vi "16chaneffective.vi"() -> ()   [LabVIEW 2013]
doc: "Cont(inuous) Acq(uire) & Chart (hw timed) demonstrates the hardware timed, non-buffered technique of data acquisition. The scan clock on the board controls acquisition timing. Acquired scans are read directly from the device's FIFO using AI Single Scan. \n\nThe acquisition is configured with no buffer, and the on-board scan clock started at the selected scan rate. In the first loop iteration, the newest (most recent) scan is read from the FIFO. In each subsequent loop iteration AI Single Scan is called to read the oldest scan from the FIFO. Then if a scan is missed because the acquisition does not keep up, an error message will be displayed, and the acquisition stopped. Each scan is plotted on the chart after it is read. \n\nA common reason to use non-buffered acquisition is that some kind of processing needs to be done for each data point. You will probably want to add more functions to the diagram to customize this VI for your application. The acquisition rate you can achieve depends on how much processing and display the VI must do. This VI calls a subVI named My Single-Scan Processing. Add whatever processing you need to this subVI, or replace it with one of your own. The data processing subVI also demonstrates how to use error clusters in your own subVIs, so they can be included in the error data flow chain.\n\nBefore running this VI, set the values of the controls on the front panel. Select Show Help Window from the Help menu to see a description of each control. If the values you select for all the controls are values you will usually use, select Make Current Values Default from the Operate menu and save the VI. Or, you may save individual control's default values by popping up on the control, selecting Data Operations, then selecting Make Current Value Default, and saving the VI."
uses:
  <vilib>/Utility/error.llb/DialogType.ctl
  <vilib>/DAQmx/read.llb/DAQmx Read (Analog 2D DBL NChan NSamp).vi
  BiaxGlobals (16chan).vi
  <vilib>/DAQmx/create/channels.llb/DAQmx Create Channel (AI-Voltage-Basic).vi
  <vilib>/DAQmx/configure/timing.llb/DAQmx Timing (Sample Clock).vi
  <vilib>/DAQmx/configure/trigger.llb/DAQmx Start Trigger (Digital Edge).vi
  effectiveglobals.vi
  <vilib>/DAQmx/miscellaneous.llb/DAQmx Fill In Error Info.vi
  <resource>/objmgr/daqmx.rc
panel:
  in  "Show plot":bool
  out "Zero Voltage Y":dbl
  in  "Calibration y-axis (V/unit)":dbl=1.0 format="%#_6f"
  in  "Select y-axis":string(combo)="Porosity"
  in  "Calibration x-axis (V/unit)":dbl=1.0 format="%#_6f"
  in  "Select x-axis":string(combo)="Time (s)"
  out "Offset Voltage 2":dbl
  out "Offset Voltage 1":dbl
  in  "Offset X-axis 2":bool
  in  "Offset X-axis 1":bool
  in  "Zero y-axis":bool
  out "XY plot":cluster{"Y":dbl[], "Y":dbl[]}[](graph)
  in  "Reset plot":bool
  out "Zero Voltage X":dbl
  in  "Zero X-axis":bool
  out "Porosity (%)":dbl format="%_4f"
  in  "Material density (g/cm3)":dbl=2.17
  in  "Amount of material (g)":dbl=42.88 format="%_4f"
  in  "Thickness (2 layers, mm)":dbl=11.28 format="%_4f"
  in  "Zero Hor DCDT":bool
  out "Average Pore pressure":dbl=0.0015205308
  out "Zeroed at:":i32
  out "Zero Voltage":dbl format="%_6g"
  in  "Zero Pore pressure A":bool
  out "Zeroed at:":i32
  out "Zero Voltage":dbl format="%_6g"
  in  "Zero Pore pressure B":bool
  out "Effective normal \nstress (MPa)":dbl=0.0015205308
  in  "Sample\n Area (m2)":dbl=0.003078
  out "Zeroed at:":i32
  out "Zero Voltage":dbl format="%_6g"
  in  "Zero Confine":bool
  in  "Horizontal Load":bool=TRUE
  out "Zeroed at:":i32
  out "Zero Voltage":dbl format="%_6g"
  in  "Zero Normal":bool
  out "Array 2":i32[][](array[numeric])=[[10000, 0, -17, -1030, -696, -422, -1063, -1097, -410, -661, -1080]]
  out "AUX8 (ch11)":dbl format="%.4f"
  out "AUX7 (ch10)":dbl format="%.4f"
  out "AUX6 (ch9)":dbl format="%.4f"
  out "AUX5 (ch8)":dbl format="%.4f"
  out "AUX4 (ch7)":dbl format="%.4f"
  out "AUX3 (ch6)":dbl format="%.4f"
  out "AUX2 (ch5)":dbl format="%.4f"
  out "AUX1 (ch4)":dbl format="%.4f"
  out "Hor Load (ch0)":dbl format="%.4f"
  out "Vert Load (ch2)":dbl format="%.4f"
  out "Hor LVDT":dbl format="%.4f"
  out "Vert LVDT (ch3)":dbl format="%.4f"
  out "Array 17":i32[][](array[numeric])=[[10000, -673, -5, -1015, -683, -421, -1049, -1100, -413, -693, -1121]]
  out "Array 16":i32[][](array[numeric])=[[10000, -673, -5, -1015, -683, -421, -1049, -1100, -413, -693, -1121]]
  out "Array 15":i32[][](array[numeric])=[[10000, -673, -5, -1015, -683, -421, -1049, -1100, -413, -693, -1121]]
  out "Array 14":i32[][](array[numeric])=[[10000, -685, -5, -1012, -680, -418, -1052, -1092, -421, -673, -1097]]
  out "AUX12 (ch15)":dbl format="%.4f"
  out "AUX11 (ch14)":dbl format="%.4f"
  out "AUX10 (ch13)":dbl format="%.4f"
  out "AUX9 (ch12)":dbl format="%.4f"
  out "element 15":string
  out "element 14":string
  out "element 13":string
  out "element 12":string
  out "element 11":string
  out "element 10":string
  out "element 9":string
  out "element 8":string
  out "element 7":string
  out "element 6":string="  "
  out "element 5":string
  out "element 4":string
  out "element 3":string
  out "element 2":string
  out "element":string
  out "element":string
  out "Stress-strain-temp vs time (Voltage)":dbl[][](graph)
  out "Array 13":i32[][](array[numeric])
  out "Array 12":i32[][](array[numeric])
  out "Array 11":i32[][](array[numeric])
  out "Array 10":i32[][](array[numeric])
  out "Array 9":i32[][](array[numeric])
  out "Array 8":i32[][](array[numeric])
  out "Array 7":i32[][](array[numeric])
  out "Array 6":i32[][](array[numeric])
  out "Array 5":i32[][](array[numeric])
  out "Array 4":i32[][](array[numeric])
  out "Array 3":i32[][](array[numeric])
  out "Array":i32[][](array[numeric])
  out "10000":bool
  in  "10 kHz":bool
  out "Processor scan rate":i32
  out "Present sample number":i32
  in  "1 Hz":bool
  out "1":bool
  out "10":bool
  out "100":bool
  out "1000":bool
  in  "10 Hz":bool
  in  "100 Hz":bool
  in  "1000 Hz":bool
  out "Data Recording Rate":i32(slide) scale=1.0..10000.0
  out "Write interval":i32
  out "Write countdown":i32
  out "Time into data acq. (s)":i32
  out "Saved sample No.":i32
  out "Record rate (samp/s)":i32
  out "No. of scans in backlog":i32
  in  "stop":bool
  # "Input Signals (volts)"
  # "To File (24 bit)"
  # "S\nI\nG\nN\nA\nL\n\nV\nO\nL\nT\nA\nG\nE"
  # "Timestamp"
  # "Data Recording Info"
  # "Acquisition Statistics"
  # "Sample (point) Number"
  # "Low gain"
  # "High gain"
  # "NOTE:  This instrument will write data (time channel then Channels 0-15) to a user defined filename.  The file is written in binary format without a header. The time channel is comprised of numbers indicating the data recording frequency (eg 1, 10, 100, 1000, 10000  samples per second)."
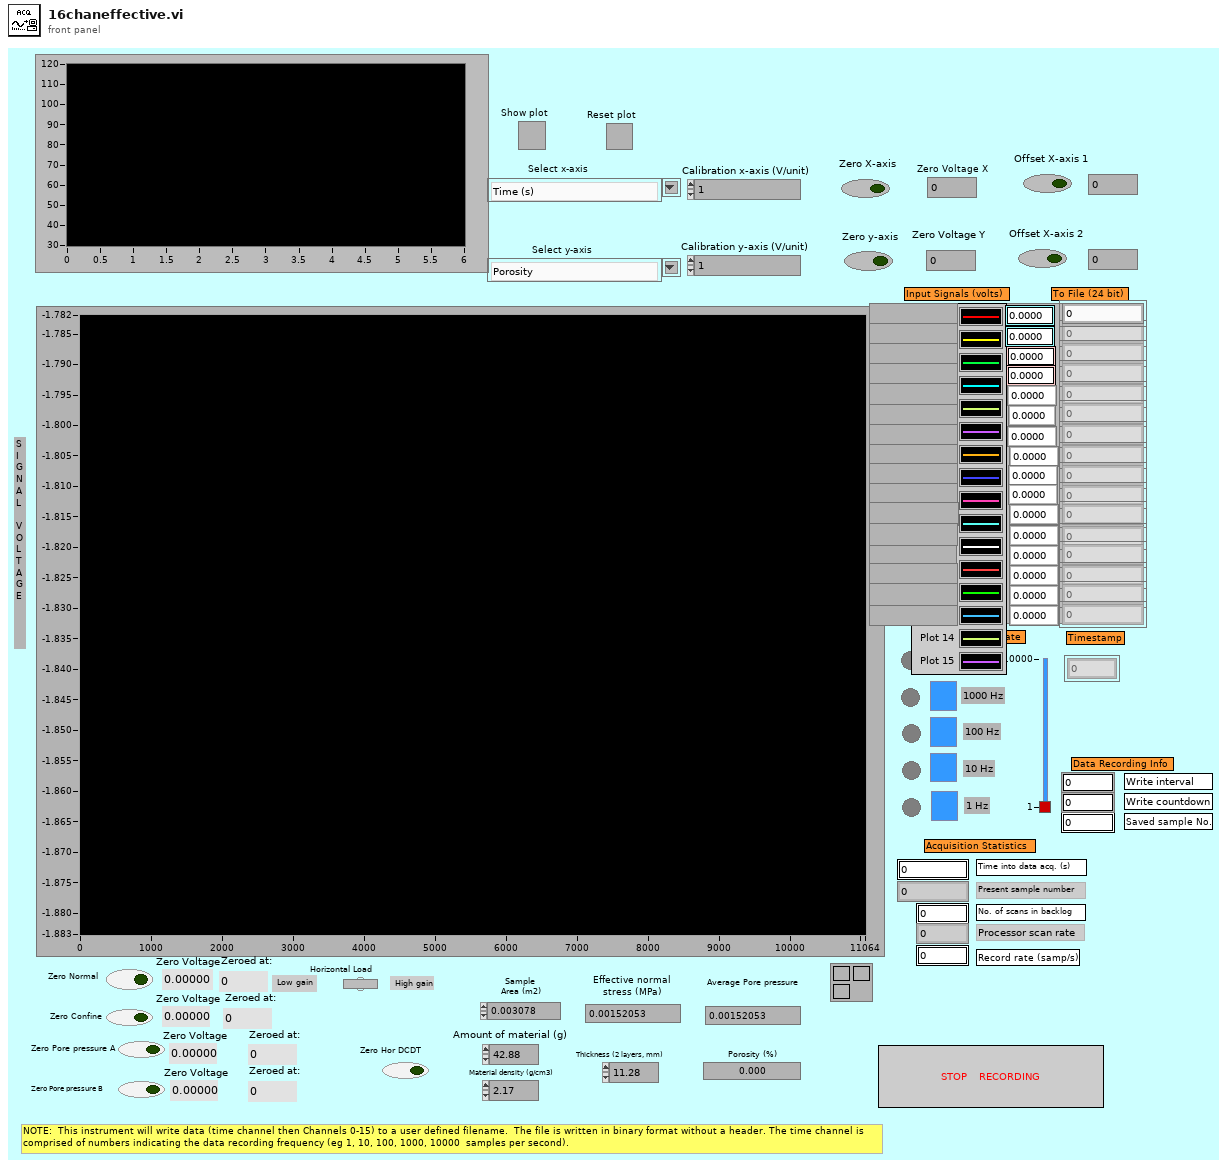
[diagram p1: front panel]
types:
  T1 = typedef "DialogType.ctl" = u16
  T2 = enum16{"big-endian, network order", "native, host order", "little-endian"}
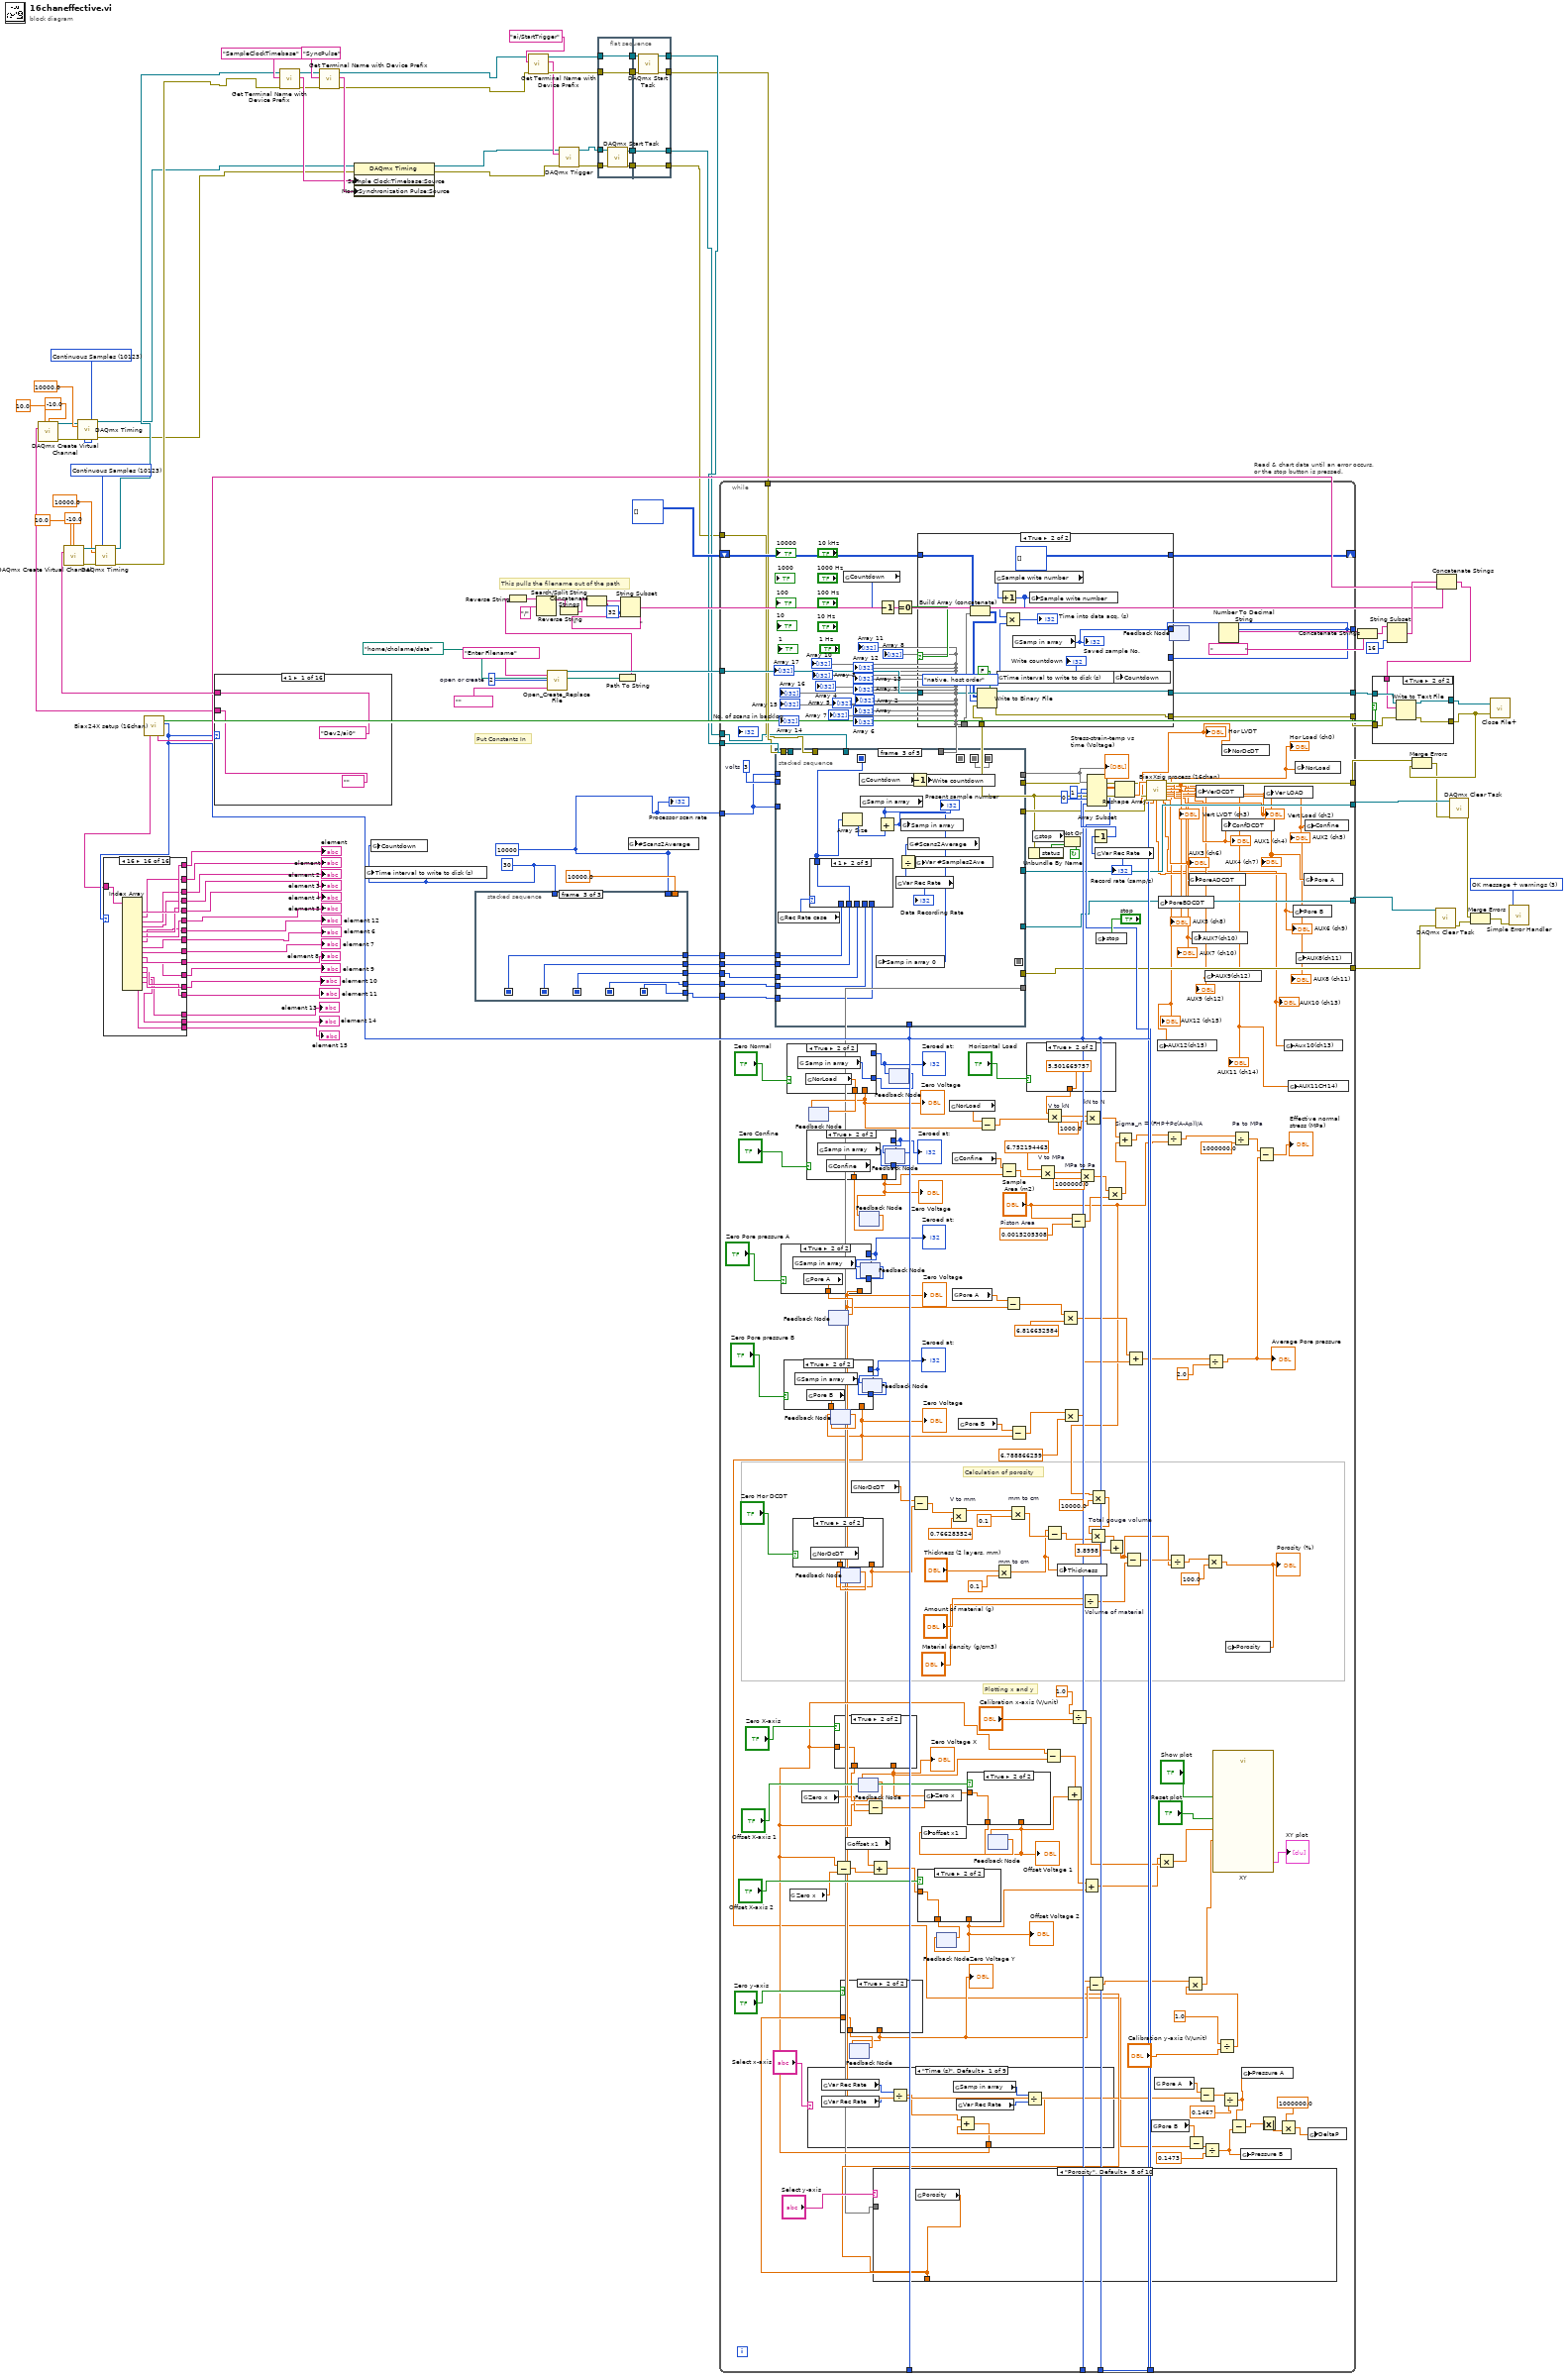
[diagram p0: block diagram]
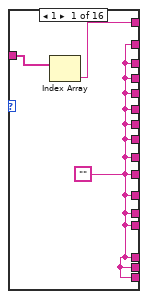
[diagram p2: hidden frame]
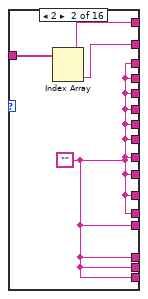
[diagram p3: hidden frame]
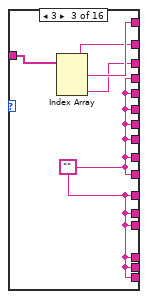
[diagram p4: hidden frame]
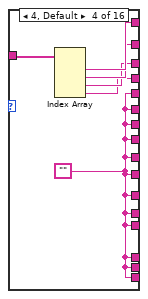
[diagram p5: hidden frame]
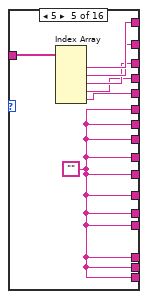
[diagram p6: hidden frame]
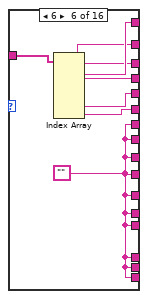
[diagram p7: hidden frame]
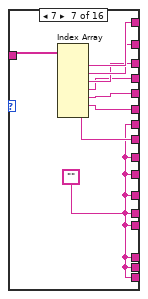
[diagram p8: hidden frame]
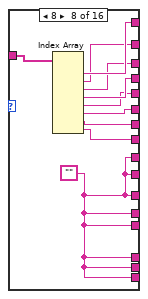
[diagram p9: hidden frame]
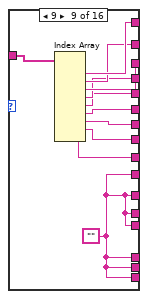
[diagram p10: hidden frame]
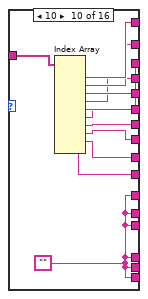
[diagram p11: hidden frame]
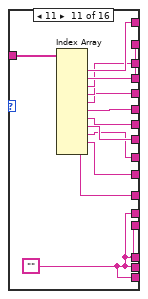
[diagram p12: hidden frame]
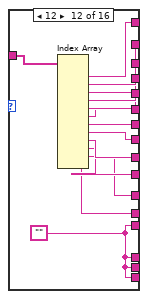
[diagram p13: hidden frame]
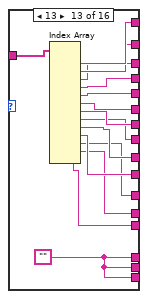
[diagram p14: hidden frame]
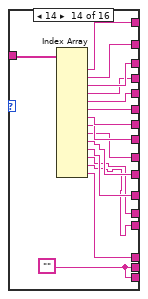
[diagram p15: hidden frame]
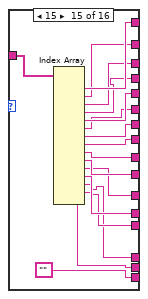
[diagram p16: hidden frame]
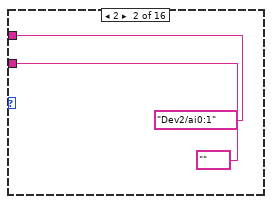
[diagram p18: hidden frame]
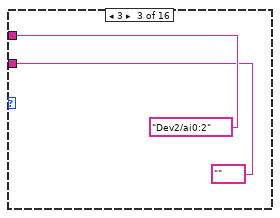
[diagram p19: hidden frame]
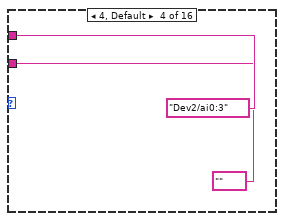
[diagram p20: hidden frame]
diagram:
  w25 = T1 3 items=["no dialog", "OK message", "continue or stop message", "OK message + warnings", "continue/stop + warnings"] ("type of dialog (OK msg:1)")
  w43 = 10123 items=["Finite Samples"=10178, "Continuous Samples"=10123, "Hardware Timed Single Point"=12522] ("sample mode")
  w30 = 10000 ("Number of scans")
  w82 = 30 ("Write time int (s)")
  w85 = 10123 items=["Finite Samples"=10178, "Continuous Samples"=10123, "Hardware Timed Single Point"=12522] ("sample mode")
  w106 = 2  # open or create
  # "This pulls the filename out of the path"
  # "Put Constants In"
  n1 = call "Biax24X setup (16chan).vi"() -> ("Footer String"=w71:string, "Number of Channels"=w65:i32, "ASCII footer 2"=w70:bool, "Channel Names"=w64:string[])  [unwired: 1 in, 4 out]
  n2 = case shown="16" w65 {
    tunnel: w64 -> [w109 w112 w117 w123 w130 w138 w147 w158 w169 w181 w194 w208 w223 w237 w254 w273]
    tunnel: [w108 w113 w118 w124 w131 w139 w148 w157 w168 w180 w193 w207 w222 w236 w255 w272] -> w53
    tunnel: [w107 w111 w116 w122 w129 w137 w146 w156 w167 w179 w192 w206 w221 w235 w253 w271] -> w63
    tunnel: [w107 w110 w115 w121 w128 w136 w145 w155 w166 w178 w191 w205 w220 w234 w252 w270] -> w62
    tunnel: [w107 w110 w114 w120 w127 w135 w144 w154 w165 w177 w190 w204 w219 w233 w251 w269] -> w61
    tunnel: [w107 w110 w114 w119 w126 w134 w143 w153 w164 w176 w189 w203 w218 w232 w250 w268] -> w60
    tunnel: [w107 w110 w114 w119 w125 w133 w142 w152 w163 w175 w188 w202 w217 w231 w249 w267] -> w59
    tunnel: [w107 w110 w114 w119 w125 w132 w141 w150 w161 w173 w186 w200 w215 w229 w247 w265] -> w58
    tunnel: [w107 w110 w114 w119 w125 w132 w140 w149 w160 w172 w185 w199 w214 w228 w246 w264] -> w57
    tunnel: [w107 w110 w114 w119 w125 w132 w140 w149 w159 w171 w184 w198 w213 w226 w245 w263] -> w56
    tunnel: [w107 w110 w114 w119 w125 w132 w140 w149 w159 w170 w183 w197 w212 w227 w244 w262] -> w55
    tunnel: [w107 w110 w114 w119 w125 w132 w140 w149 w159 w170 w182 w196 w211 w225 w243 w261] -> w54
    tunnel: [w107 w110 w114 w119 w125 w132 w140 w149 w159 w170 w182 w195 w210 w224 w242 w260] -> w52
    tunnel: [w107 w110 w114 w119 w125 w132 w140 w149 w159 w170 w182 w195 w209 w238 w241 w259] -> w51
    tunnel: [w107 w110 w114 w119 w125 w132 w140 w149 w159 w170 w182 w195 w209 w239 w240 w258] -> w50
    tunnel: [w107 w110 w114 w119 w125 w132 w140 w149 w159 w170 w182 w195 w209 w239 "" w257] -> w49
    tunnel: [w107 w110 w114 w119 w125 w132 w140 w151 w162 w174 w187 w201 w216 w230 w248 w266] -> w48
    frame 1 {
      w107 = ""
      n3 = Index Array(array=w109) -> (element=w108:string)  [unwired: 1 in]
    }
    frame 2 {
      w110 = ""
      n4 = Index Array(array=w112) -> (element #1=w113:string, element #2=w111:string)  [unwired: 2 in]
    }
    frame 3 {
      w114 = ""
      n5 = Index Array(array=w117) -> (element #1=w118:string, element #2=w116:string, element #3=w115:string)  [unwired: 3 in]
    }
    frame 4, Default {
      w119 = ""
      n6 = Index Array(array=w123) -> (element #1=w124:string, element #2=w122:string, element #3=w121:string, element #4=w120:string)  [unwired: 4 in]
    }
    frame 5 {
      w125 = ""
      n7 = Index Array(array=w130) -> (element #1=w131:string, element #2=w129:string, element #3=w128:string, element #4=w127:string, element #5=w126:string)  [unwired: 5 in]
    }
    frame 6 {
      w132 = ""
      n8 = Index Array(array=w138) -> (element #1=w139:string, element #2=w137:string, element #3=w136:string, element #4=w135:string, element #5=w134:string, element #6=w133:string)  [unwired: 6 in]
    }
    frame 7 {
      w140 = ""
      n9 = Index Array(array=w147) -> (element #1=w148:string, element #2=w146:string, element #3=w145:string, element #4=w144:string, element #5=w143:string, element #6=w142:string, element #7=w141:string)  [unwired: 7 in]
    }
    frame 8 {
      w149 = ""
      n10 = Index Array(array=w158) -> (element #1=w157:string, element #2=w156:string, element #3=w155:string, element #4=w154:string, element #5=w153:string, element #6=w152:string, element #7=w151:string, element #8=w150:string)  [unwired: 8 in]
    }
    frame 9 {
      w159 = ""
      n11 = Index Array(array=w169) -> (element #1=w168:string, element #2=w167:string, element #3=w166:string, element #4=w165:string, element #5=w164:string, element #6=w163:string, element #7=w162:string, element #8=w161:string, element #9=w160:string)  [unwired: 9 in]
    }
    frame 10 {
      w170 = ""
      n12 = Index Array(array=w181) -> (element #1=w180:string, element #2=w179:string, element #3=w178:string, element #4=w177:string, element #5=w176:string, element #6=w175:string, element #7=w174:string, element #8=w173:string, element #9=w172:string, element #10=w171:string)  [unwired: 10 in]
    }
    frame 11 {
      w182 = ""
      n13 = Index Array(array=w194) -> (element #1=w193:string, element #2=w192:string, element #3=w191:string, element #4=w190:string, element #5=w189:string, element #6=w188:string, element #7=w187:string, element #8=w186:string, element #9=w185:string, element #10=w184:string, element #11=w183:string)  [unwired: 11 in]
    }
    frame 12 {
      w195 = ""
      n14 = Index Array(array=w208) -> (element #1=w207:string, element #2=w206:string, element #3=w205:string, element #4=w204:string, element #5=w203:string, element #6=w202:string, element #7=w201:string, element #8=w200:string, element #9=w199:string, element #10=w198:string, element #11=w197:string, element #12=w196:string)  [unwired: 12 in]
    }
    frame 13 {
      w209 = ""
      n15 = Index Array(array=w223) -> (element #1=w222:string, element #2=w221:string, element #3=w220:string, element #4=w219:string, element #5=w218:string, element #6=w217:string, element #7=w216:string, element #8=w215:string, element #9=w214:string, element #10=w213:string, element #11=w212:string, element #12=w211:string, element #13=w210:string)  [unwired: 13 in]
    }
    frame 14 {
      w239 = ""
      n16 = Index Array(array=w237) -> (element #1=w236:string, element #2=w235:string, element #3=w234:string, element #4=w233:string, element #5=w232:string, element #6=w231:string, element #7=w230:string, element #8=w229:string, element #9=w228:string, element #10=w226:string, element #11=w227:string, element #12=w225:string, element #13=w224:string, element #14=w238:string)  [unwired: 14 in]
    }
    frame 15 {
      n17 = Index Array(array=w254) -> (element #1=w255:string, element #2=w253:string, element #3=w252:string, element #4=w251:string, element #5=w250:string, element #6=w249:string, element #7=w248:string, element #8=w247:string, element #9=w246:string, element #10=w245:string, element #11=w244:string, element #12=w243:string, element #13=w242:string, element #14=w241:string, element #15=w240:string)  [unwired: 15 in]
    }
    frame 16 {
      n18 = Index Array(array=w273) -> (element #1=w272:string, element #2=w271:string, element #3=w270:string, element #4=w269:string, element #5=w268:string, element #6=w267:string, element #7=w266:string, element #8=w265:string, element #9=w264:string, element #10=w263:string, element #11=w262:string, element #12=w261:string, element #13=w260:string, element #14=w259:string, element #15=w258:string, element #16=w257:string)  [unwired: 16 in]
    }
  }
  "element" <- w53
  "element" <- w63
  "element 2" <- w62
  "element 3" <- w61
  "element 4" <- w60
  "element 5" <- w59
  "element 6" <- w58
  "element 7" <- w57
  "element 8" <- w56
  "element 9" <- w55
  "element 10" <- w54
  "element 11" <- w52
  "element 12" <- w48
  "element 13" <- w51
  "element 14" <- w50
  "element 15" <- w49
  n19 = case shown="1" w65 {
    tunnel: [tag "Dev2/ai0" ("physical channels") tag "Dev2/ai0:1" ("physical channels") tag "Dev2/ai0:2" ("physical channels") tag "Dev2/ai0:3" ("physical channels") tag "Dev2/ai0:4" ("physical channels") tag "Dev2/ai0:5" ("physical channels") tag "Dev2/ai0:6" ("physical channels") tag "Dev2/ai0:7" ("physical channels") tag "Dev2/ai0:7" ("physical channels") tag "Dev2/ai0:7" ("physical channels") tag "Dev2/ai0:7" ("physical channels") tag "Dev2/ai0:7" ("physical channels") tag "Dev2/ai0:7" ("physical channels") tag "Dev2/ai0:7" ("physical channels") tag "Dev2/ai0:7" ("physical channels") tag "Dev2/ai0:7" ("physical channels")] -> w79
    tunnel: [tag "" ("physical channels") tag "" ("physical channels") tag "" ("physical channels") tag "" ("physical channels") tag "" ("physical channels") tag "" ("physical channels") tag "" ("physical channels") tag "" ("physical channels") tag "Dev1/ai0" ("physical channels") tag "Dev1/ai0:1" ("physical channels") tag "Dev1/ai0:2" ("physical channels") tag "Dev1/ai0:3" ("physical channels") tag "Dev1/ai0:4" ("physical channels") tag "Dev1/ai0:5" ("physical channels") tag "Dev1/ai0:6" ("physical channels") tag "Dev1/ai0:7" ("physical channels")] -> w47
    frame 1 {
    }
    frame 2 {
    }
    frame 3 {
    }
    frame 4, Default {
    }
    frame 5 {
    }
    frame 6 {
    }
    frame 7 {
    }
    frame 8 {
    }
    frame 9 {
    }
    frame 10 {
    }
    frame 11 {
    }
    frame 12 {
    }
    frame 13 {
    }
    frame 14 {
    }
    frame 15 {
    }
    frame 16 {
    }
  }
  n20 = call-poly <vilib>:"DAQmx Create Virtual Channel.vi"("maximum value"=10.0, "minimum value"=-10.0, "physical channels"=w47) -> ("task out"=w42:refnum<k21>, "error out"=w41:errorcluster)  [unwired: 11 in]
  n21 = call-poly <vilib>:"DAQmx Create Virtual Channel.vi"("maximum value"=10.0, "minimum value"=-10.0, "physical channels"=w79) -> ("task out"=w87:refnum<k21>, "error out"=w86:errorcluster)  [unwired: 11 in]
  n22 = call-poly <vilib>:"DAQmx Timing.vi"("task/channels in"=w42, "sample mode"=w43, "rate"=10000.0, "error in"=w41) -> ("task out"=w4:refnum<k21>, "error out"=w5:errorcluster)  [unwired: 10 in]
  n23 = call-poly <vilib>:"DAQmx Timing.vi"("task/channels in"=w87, "sample mode"=w85, "rate"=10000.0, "error in"=w86) -> ("task out"=w9:refnum<k21>, "error out"=w8:errorcluster)  [unwired: 10 in]
  n24 = call "Get Terminal Name with Device Prefix.vi"("error in"=w8, "Local Terminal Name"="SampleClockTimebase", "task/channels in"=w9) -> ("error out"=w13:errorcluster, "Terminal Name with Device Prefix"=w14:tag, "task out"=w11:refnum<k21>)  [unwired: 6 in]
  n25 = call "Get Terminal Name with Device Prefix.vi"("error in"=w13, "Local Terminal Name"="SyncPulse", "task/channels in"=w11) -> ("error out"=w6:errorcluster, "Terminal Name with Device Prefix"=w15:tag, "task out"=w7:refnum<k21>)  [unwired: 6 in]
  n26 = property class="DAQmx Timing"(reference=w4, error in=w5, "Sample Clock:Timebase:Source"=w14, "More:Synchronization Pulse:Source"=w15) -> (reference out=w3:refnum<k21>, error out=w2:errorcluster)
  n27 = global write "BiaxGlobals (16chan).vi" "Time interval to write to disk (s)"(w82) -> ()
  n28 = global write "BiaxGlobals (16chan).vi" "Countdown"(w82) -> ()
  n29 = stacked-sequence {
    seq-local: [_ w326 _] -> [_ _ w339]
    seq-local: [_ w323 _] -> [_ _ w336]
    seq-local: [_ w318 _] -> [_ _ w338]
    seq-local: [_ w317 _] -> [_ _ w337]
    seq-local: [_ w312 _] -> [_ _ w335]
    tunnel: w82 -> [w306 _ _]
    tunnel: w30 -> [w310 _ _]
    tunnel: sgl 10000.0 ("actual scan rate") -> [w308 _ _]
    tunnel: [_ _ w339] -> w101
    tunnel: [_ _ w336] -> w100
    tunnel: [_ _ w338] -> w99
    tunnel: [_ _ w337] -> w98
    tunnel: [_ _ w335] -> w97
    frame #0 {
      w307 = i16 0
      n30 = local write "Time into data acq. (s)"(w307) -> ()
      n31 = global write "BiaxGlobals (16chan).vi" "Sample write number"(w307) -> ()
      n32 = global write "BiaxGlobals (16chan).vi" "Time interval to write to disk (s)"(w306) -> ()
      n33 = Divide(x=w308, y=w310) -> (x/y=w309:sgl)
      n34 = global write "BiaxGlobals (16chan).vi" "Rec Rate (samp/s)"(w309) -> ()
      n35 = local write "Write countdown"(w306) -> ()
      n36 = local write "Saved sample No."(w307) -> ()
      n37 = global write "BiaxGlobals (16chan).vi" "Samp in array"(w307) -> ()
    }
    frame #1 {
      n38 = Initialize Array(i16 1, 10000) -> (w326:i16[])
      n39 = global write "BiaxGlobals (16chan).vi" "Rec Rate case"(4) -> ()
      n40 = local write "10"(FALSE) -> ()
      n41 = local write "1"(TRUE) -> ()
      n42 = Initialize Array(i16 10, 1000) -> (w323:i16[])
      n43 = local write "1000"(FALSE) -> ()
      n44 = local write "100"(FALSE) -> ()
      n45 = global read "BiaxGlobals (16chan).vi" "Time interval to write to disk (s)"() -> (→"Write interval":i32)
      n46 = Initialize Array(i16 100, 100) -> (w318:i16[])
      n47 = local write "10000"(FALSE) -> ()
      n48 = Initialize Array(i16 1000, 10) -> (w317:i16[])
      n49 = Initialize Array(i16 10000, 1) -> (w312:i16[])
      n50 = global write "BiaxGlobals (16chan).vi" "Accum Time"(0) -> ()
      n51 = global write "BiaxGlobals (16chan).vi" "Var Rec Rate"(1) -> ()
    }
    frame #2 {
    }
  }
  n52 = call "Get Terminal Name with Device Prefix.vi"("error in"=w6, "Local Terminal Name"="ai/StartTrigger" ("terminal"), "task/channels in"=w7) -> ("error out"=w32:errorcluster, "Terminal Name with Device Prefix"=w31:tag, "task out"=w35:refnum<k21>)  [unwired: 6 in]
  n53 = call <vilib>:"Open_Create_Replace File.vi"("default name"="", "prompt"="Enter Filename", "function (open:0)"=w106, "start path  (Not A Path)"=path "/home/cholame/data") -> ("new file path"=w96:path, "refnum"=w103:refnum<file>)  [unwired: 4 in, 2 out]
  n54 = call-poly <vilib>:"DAQmx Trigger.vi"("task/channels in"=w3, "source"=w31, "error in"=w2) -> ("task out"=w34:refnum<k21>, "error out"=w33:errorcluster)  [unwired: 11 in]
  n55 = flat-sequence {
    tunnel: w34 -> [w344]
    tunnel: w33 -> [w343]
    tunnel: [w345] -> w40
    tunnel: w35 -> [w342]
    tunnel: [w342] -> w39
    tunnel: [w341] -> w38
    tunnel: w32 -> [w341]
    tunnel: [w340] -> w37
    tunnel: [w351] -> w27
    tunnel: w40 -> [w351]
    tunnel: w39 -> [w350]
    tunnel: w38 -> [w349]
    tunnel: [w348] -> w28
    tunnel: [w347] -> w29
    tunnel: [w346] -> w26
    tunnel: w37 -> [w346]
    frame #0 {
      n56 = call <vilib>:"DAQmx Start Task.vi"("task/channels in"=w344, "error in"=w343) -> ("task out"=w345:refnum<k21>, "error out"=w340:errorcluster)  [unwired: 12 in]
    }
    frame #1 {
      n57 = call <vilib>:"DAQmx Start Task.vi"("task/channels in"=w350, "error in"=w349) -> ("task out"=w347:refnum<k21>, "error out"=w348:errorcluster)  [unwired: 12 in]
    }
  }
  n58 = Path To String(path=w96) -> (string=w93:string)
  n59 = Reverse String(1:w93) -> (0:w94:string)
  n60 = Search/Split String(string=w94, search string/char (-)="/") -> (substring before match=w92:string)  [unwired: 1 in, 2 out]
  n61 = Reverse String(1:w92) -> (0:w88:string)
  n62 = Concatenate Strings(w88, "                                ") -> (w90:string)
  n63 = String Subset(string=w90, length (rest)=32 ("length (rest)")) -> (substring=w72:string)  [unwired: 1 in]
  n64 = global write "BiaxGlobals (16chan).vi" "#Scans2Average"(w30) -> ()
  n65 = while "Read & chart data until an error occurs,\nor the stop button is pressed." {
    tunnel: w97 -> [w517]
    tunnel: w98 -> [w519]
    tunnel: w99 -> [w520]
    tunnel: w100 -> [w521]
    tunnel: w101 -> [w522]
    shift-left: i16[][] [] -> [w509]
    shift-right: [w535] -> _
    tunnel: w30 -> [w523]
    tunnel: [w536] -> w67
    tunnel: [w537] -> w69
    tunnel: w103 -> [w538]
    tunnel: w65 -> [w516]
    tunnel: w65 -> [w510]
    tunnel: w65 -> [w515]
    tunnel: w65 -> [w511]
    tunnel: [w507] -> w78
    tunnel: w29 -> [w503]
    tunnel: w28 -> [w502]
    tunnel: w27 -> [w501]
    tunnel: w26 -> [w500]
    tunnel: [w499] -> w22
    tunnel: [w498] -> w18
    tunnel: [w497] -> w21
    tunnel: [w496] -> w20
    stop <- w534 continue-if-true
    w458 = 0.0015205308  # Piston Area
    w529 = 3  # volts
    # "Plotting x and y"
    # "Calculation of porosity"
    n66 = stacked-sequence {
      seq-local: [_ _ w661 _ _] -> [_ _ _ _ w703]
      seq-local: [_ _ _ w679 _] -> [_ _ _ _ w700]
      seq-local: [w616 _ _ _ _] -> [_ w630 _ _ _]
      seq-local: [_ w630 _ _ _] -> [_ _ w659 _ _]
      seq-local: [_ _ w659 _ _] -> [_ _ _ w678 _]
      tunnel: w529 -> [_ _ _ _ _]
      tunnel: w523 -> [_ _ _ w682 _]
      tunnel: [w620 _ _ _ _] -> w513
      tunnel: [_ _ _ _ w700] -> w506
      tunnel: w523 -> [w629 _ _ _ w708]
      tunnel: w522 -> [_ _ w669 _ _]
      tunnel: w521 -> [_ _ w668 _ _]
      tunnel: w520 -> [_ _ w667 _ _]
      tunnel: w519 -> [_ _ w666 _ _]
      tunnel: [_ _ _ _ w702] -> w504
      tunnel: w517 -> [_ _ w660 _ _]
      tunnel: w515 -> [_ _ _ w680 _]
      tunnel: w502 -> [w627 _ _ _ _]
      tunnel: w503 -> [w628 _ _ _ _]
      tunnel: w501 -> [w626 _ _ _ _]
      tunnel: w500 -> [w625 _ _ _ _]
      tunnel: [w621 _ _ _ _] -> w499
      tunnel: [w622 _ _ _ _] -> w498
      tunnel: [w619 _ _ _ _] -> w497
      tunnel: [w618 _ _ _ _] -> w496
      tunnel: [_ _ _ _ w700] -> w371
      frame #0 {
        n67 = call-poly <vilib>:"DAQmx Read.vi"("task/channels in"=w626, "number of samples per channel"=w629, "error in"=w625) -> ("task out"=w618:refnum<k21>, "data"=w623:dbl[][], "error out"=w621:errorcluster)  [unwired: 10 in]
        n68 = call-poly <vilib>:"DAQmx Read.vi"("task/channels in"=w628, "number of samples per channel"=w629, "error in"=w627) -> ("task out"=w619:refnum<k21>, "data"=w624:dbl[][], "error out"=w622:errorcluster)  [unwired: 10 in]
        n69 = Insert Into Array(array=w624, new element=w623) -> (w617:dbl[][])  [unwired: 2 in]
        n70 = Transpose 2D Array(2D array=w617) -> (transposed array=w616:dbl[][])
        n71 = Merge Errors(w622, w621) -> (w620:errorcluster)
      }
      frame #1 {
        n72 = local read "1000 Hz"() -> (w635:bool)
        n73 = local read "100 Hz"() -> (w634:bool)
        n74 = local read "10 Hz"() -> (w633:bool)
        n75 = local read "1 Hz"() -> (w632:bool)
        n76 = local read "10 kHz"() -> (w631:bool)
        n77 = case shown="True" w631 {
          frame False {
          }
          frame True {
            w636 = FALSE
            n78 = local write "1"(w636) -> ()
            n79 = local write "10"(w636) -> ()
            n80 = local write "100"(w636) -> ()
            n81 = local write "1000"(w636) -> ()
            n82 = local write "10000"(TRUE ("10x")) -> ()
            n83 = global write "BiaxGlobals (16chan).vi" "Rec Rate case"(0) -> ()
            n84 = global write "BiaxGlobals (16chan).vi" "Var Rec Rate"(10000) -> ()
          }
        }
        n85 = case shown="True" w635 {
          frame False {
          }
          frame True {
            w652 = FALSE
            n86 = local write "1"(w652) -> ()
            n87 = local write "10"(w652) -> ()
            n88 = local write "100"(w652) -> ()
            n89 = local write "10000"(w652) -> ()
            n90 = local write "1000"(TRUE ("10x")) -> ()
            n91 = global write "BiaxGlobals (16chan).vi" "Rec Rate case"(1) -> ()
            n92 = global write "BiaxGlobals (16chan).vi" "Var Rec Rate"(1000) -> ()
          }
        }
        n93 = case shown="True" w634 {
          frame False {
          }
          frame True {
            w648 = FALSE
            n94 = local write "1"(w648) -> ()
            n95 = local write "10"(w648) -> ()
            n96 = local write "1000"(w648) -> ()
            n97 = local write "10000"(w648) -> ()
            n98 = local write "100"(TRUE ("1x")) -> ()
            n99 = global write "BiaxGlobals (16chan).vi" "Rec Rate case"(2) -> ()
            n100 = global write "BiaxGlobals (16chan).vi" "Var Rec Rate"(100) -> ()
          }
        }
        n101 = case shown="True" w633 {
          frame False {
          }
          frame True {
            w644 = FALSE
            n102 = local write "1"(w644) -> ()
            n103 = local write "100"(w644) -> ()
            n104 = local write "1000"(w644) -> ()
            n105 = local write "10000"(w644) -> ()
            n106 = local write "10"(TRUE ("0.1x")) -> ()
            n107 = global write "BiaxGlobals (16chan).vi" "Rec Rate case"(3) -> ()
            n108 = global write "BiaxGlobals (16chan).vi" "Var Rec Rate"(10) -> ()
          }
        }
        n109 = case shown="True" w632 {
          frame False {
          }
          frame True {
            w640 = FALSE
            n110 = local write "10"(w640) -> ()
            n111 = local write "100"(w640) -> ()
            n112 = local write "1000"(w640) -> ()
            n113 = local write "10000"(w640) -> ()
            n114 = local write "1"(TRUE) -> ()
            n115 = global write "BiaxGlobals (16chan).vi" "Rec Rate case"(4) -> ()
            n116 = global write "BiaxGlobals (16chan).vi" "Var Rec Rate"(1) -> ()
          }
        }
      }
      frame #2 {
        n117 = global read "BiaxGlobals (16chan).vi" "Rec Rate case"() -> (w665:i32)
        n118 = case shown="1" w665 {
          tunnel: w669 -> [w672 _ _ _ _]
          tunnel: [w672 w673 w674 w675 w676] -> w661
          tunnel: w668 -> [_ w673 _ _ _]
          tunnel: w667 -> [_ _ w674 _ _]
          tunnel: w666 -> [_ _ _ w675 _]
          tunnel: w660 -> [_ _ _ _ w676]
          frame ..0 {
          }
          frame 1 {
          }
          frame 2 {
          }
          frame 3 {
          }
          frame 4.. {
          }
        }
        n119 = Array Size(array=w661) -> (size(s)=w664:i32)
        n120 = global read "BiaxGlobals (16chan).vi" "Countdown"() -> (w663:i32)
        n121 = global read "BiaxGlobals (16chan).vi" "Samp in array"() -> (w656:i32)
        n122 = global write "BiaxGlobals (16chan).vi" "Samp in array 0"(w656) -> ()
        n123 = Add(x=w656, y=w664) -> (x+y=w658:i32)
        "Present sample number" <- w658
        n124 = global read "BiaxGlobals (16chan).vi" "Var Rec Rate"() -> (w657:i32)
        "Data Recording Rate" <- w657
        n125 = global write "BiaxGlobals (16chan).vi" "Samp in array"(w658) -> ()
        n126 = global read "BiaxGlobals (16chan).vi" "#Scans2Average"() -> (w671:i16)
        n127 = Divide(x=w671, y=w657) -> (x/y=w670:dbl)
        n128 = Decrement(x=w663) -> (x-1=w662:i32)
        n129 = global write "BiaxGlobals (16chan).vi" "Var #Samples2Ave"(w670) -> ()
        n130 = local write "Write countdown"(w662) -> ()
      }
      frame #3 {
        n131 = To Long Integer(number=w682) -> (32bit integer=w681:i32)
        n132 = global read "BiaxGlobals (16chan).vi" "Var Rec Rate"() -> (w683:i32)
        n133 = Equal?(x=w683, y=w681) -> (x = y?=w677:bool)
        n134 = case shown="False" w677 {
          tunnel: w680 -> [w687 _]
          tunnel: w678 -> [w686 w699]
          tunnel: [w684 w699] -> w679
          frame False {
            n135 = global read "BiaxGlobals (16chan).vi" "Var Rec Rate"() -> (w688:i32)
            n136 = for {
              N: w688 -> [_]
              tunnel: w687 -> [w695]
              tunnel: w686 -> [w693]
              shift-right: [w689] -> w684
              shift-left: dbl[][] [] -> [w690]
              i -> [w698]
              n137 = global read "BiaxGlobals (16chan).vi" "Var #Samples2Ave"() -> (w694:i32)
              n138 = Multiply(x=w694, y=w698) -> ()  [unwired: 1 out]
              n139 = Multiply(x=w694, y=w698) -> (x*y=w696:i32)
              n140 = Array Subset(array=w693, index (row)=w696, length (row)=w694, index (col)=i16 0, length (col)=w695) -> (w692:dbl[][])
              n141 = call "Average Signal Voltage v(16chan).vi"("voltage data"=w692) -> ("average value\nper channel"=w691:dbl[])  [unwired: 2 in]
              n142 = Build Array (concatenate)(w690, w691) -> (w689:dbl[][])
            }
          }
          frame True {
          }
        }
      }
      frame #4 {
        (unwired) 1000.0
        n143 = global read "BiaxGlobals (16chan).vi" "Accum Time"() -> (w710:dbl)
        n144 = Transpose 2D Array(2D array=w700) -> (transposed array=w707:dbl[][])
        n145 = Multiply(x=838860.8, y=w707) -> (x*y=w705:dbl[][])
        n146 = To Long Integer(number=w705) -> (32bit integer=w704:i32[][])
        n147 = Add(x=w708, y=w710) -> (x+y=w709:dbl)
        n148 = Build Array (concatenate)(w703, w704) -> (w701:i32[][])
        n149 = Transpose 2D Array(2D array=w701) -> (transposed array=w702:i32[][])
        n150 = global write "BiaxGlobals (16chan).vi" "Accum Time"(w709) -> ()
      }
    }
    "Stress-strain-temp vs time (Voltage)" <- w506
    "Array" <- w504
    "Array 3" <- w504
    "Array 4" <- w504
    "Array 5" <- w504
    "Array 6" <- w504
    "Array 7" <- w504
    "Array 8" <- w504
    "Array 9" <- w504
    "Array 10" <- w504
    "Array 11" <- w504
    "Array 12" <- w504
    "Array 13" <- w504
    "Array 14" <- w504
    "Array 15" <- w504
    "Array 16" <- w504
    "Array 17" <- w504
    "Array 2" <- w504
    n151 = global read "effectiveglobals.vi" "Zero x"() -> (w375:dbl)
    n152 = global read "effectiveglobals.vi" "Zero x"() -> (w382:dbl)
    n153 = case shown="\"Time (s)\", Default" "Select x-axis" {
      tunnel: [w573 w580 w581 w582 w583 w584 w585 w586 w587] -> w376
      frame "Time (s)", Default {
        n154 = global read "BiaxGlobals (16chan).vi" "Var Rec Rate"() -> (w579:i32)
        n155 = global read "BiaxGlobals (16chan).vi" "Var Rec Rate"() -> (w578:i32)
        n156 = Divide(x=w579, y=w578) -> (x/y=w574:dbl)
        n157 = global read "BiaxGlobals (16chan).vi" "Samp in array"() -> (w577:i32)
        n158 = global read "BiaxGlobals (16chan).vi" "Var Rec Rate"() -> (w576:i32)
        n159 = Divide(x=w577, y=w576) -> (x/y=w575:dbl)
        n160 = Add(x=w574, y=w575) -> (x+y=w573:dbl)
      }
      frame "LP displacement" {
        n161 = global read "effectiveglobals.vi" "VerDCDT"() -> (w580:dbl)
      }
      frame "Shear load" {
        n162 = global read "effectiveglobals.vi" "Ver LOAD"() -> (w581:dbl)
      }
      frame "Normal displacement" {
        n163 = global read "effectiveglobals.vi" "NorDcDT"() -> (w582:dbl)
      }
      frame "Normal load" {
        n164 = global read "effectiveglobals.vi" "NorLoad"() -> (w583:dbl)
      }
      frame "Pore pressure A displacement" {
        n165 = global read "effectiveglobals.vi" "PoreADCDT"() -> (w584:dbl)
      }
      frame "Pore pressure A" {
        n166 = global read "effectiveglobals.vi" "Pore A"() -> (w585:dbl)
      }
      frame "Pore Preesure B Displacement" {
        n167 = global read "effectiveglobals.vi" "PoreBDCDT"() -> (w586:dbl)
      }
      frame "Pore Pressure B" {
        n168 = global read "effectiveglobals.vi" "Pore B"() -> (w587:dbl)
      }
    }
    n169 = feedback #1() -> (w474:dbl)  [unwired: 1 in]
    "Zero Voltage" <- w474
    n170 = feedback #2() -> (w356:dbl)  [unwired: 1 in]
    "Zero Voltage" <- w356
    n171 = feedback #3() -> (w355:dbl)  [unwired: 1 in]
    "Zero Voltage" <- w355
    n172 = Subtract(x=w376, y=w375) -> (x-y=w374:dbl)
    n173 = feedback #4() -> (w414:dbl)  [unwired: 1 in]
    n174 = case shown="True" "Zero Hor DCDT" {
      tunnel: [w596 w597] -> w427
      tunnel: w414 -> [w596 _]
      frame False {
      }
      frame True {
        n175 = global read "effectiveglobals.vi" "NorDcDT"() -> (w597:dbl)
      }
    }
    n176 = feedback-in #4(w427) -> ()
    n177 = global read "BiaxGlobals (16chan).vi" "Countdown"() -> (w518:i32)
    n178 = global read "effectiveglobals.vi" "offset x1"() -> (w373:dbl)
    n179 = feedback #5() -> (w390:dbl)  [unwired: 1 in]
    "Zero Voltage Y" <- w390
    n180 = global read "effectiveglobals.vi" "NorDcDT"() -> (w415:dbl)
    n181 = feedback #6() -> (w384:dbl)  [unwired: 1 in]
    "Zero Voltage X" <- w384
    n182 = case shown="True" "Zero X-axis" {
      tunnel: [w594 w595] -> w388
      tunnel: w376 -> [_ w595]
      tunnel: w384 -> [w594 _]
      frame False {
      }
      frame True {
      }
    }
    n183 = feedback-in #6(w388) -> ()
    n184 = feedback #7() -> (w464:dbl)  [unwired: 1 in]
    "Zero Voltage" <- w464
    n185 = feedback #8() -> (w447:i32)  [unwired: 1 in]
    "Zeroed at:" <- w447
    n186 = case shown="True" "Zero Pore pressure A" {
      tunnel: [w603 w605] -> w448
      tunnel: [w602 w604] -> w449
      tunnel: w356 -> [w602 _]
      tunnel: w447 -> [w603 _]
      frame False {
      }
      frame True {
        n187 = global read "BiaxGlobals (16chan).vi" "Samp in array"() -> (w605:i32)
        n188 = global read "effectiveglobals.vi" "Pore A"() -> (w604:dbl)
      }
    }
    n189 = feedback-in #2(w449) -> ()
    n190 = feedback-in #8(w448) -> ()
    n191 = feedback #9() -> (w444:i32)  [unwired: 1 in]
    "Zeroed at:" <- w444
    n192 = case shown="True" "Zero Pore pressure B" {
      tunnel: [w599 w601] -> w445
      tunnel: [w598 w600] -> w446
      tunnel: w355 -> [w598 _]
      tunnel: w444 -> [w599 _]
      frame False {
      }
      frame True {
        n193 = global read "BiaxGlobals (16chan).vi" "Samp in array"() -> (w601:i32)
        n194 = global read "effectiveglobals.vi" "Pore B"() -> (w600:dbl)
      }
    }
    n195 = feedback-in #3(w446) -> ()
    n196 = feedback-in #9(w445) -> ()
    n197 = Subtract(x=w376, y=w382) -> (x-y=w381:dbl)
    n198 = Add(x=w373, y=w374) -> (x+y=w372:dbl)
    n199 = case shown="\"Porosity\", Default" "Select y-axis" {
      tunnel: [w539 w540 w541 w542 w552 w568 w569 w570 w571 w572] -> w389
      tunnel: w371 -> [_ _ _ _ w561 _ _ _ _ _]
      frame "Shear load" {
        n200 = global read "effectiveglobals.vi" "Ver LOAD"() -> (w539:dbl)
      }
      frame "Normal displacement" {
        n201 = global read "effectiveglobals.vi" "NorDcDT"() -> (w540:dbl)
      }
      frame "Normal load" {
        n202 = global read "effectiveglobals.vi" "NorLoad"() -> (w541:dbl)
      }
      frame "Pore pressure A displacement" {
        n203 = global read "effectiveglobals.vi" "PoreADCDT"() -> (w542:dbl)
      }
      frame "Permeability A" {
        n204 = Array Subset(array=w561, index (row)=0 ("index"), length (row)=1 ("index")) -> (w566:dbl[][])  [unwired: 2 in]
        n205 = global read "BiaxGlobals (16chan).vi" "Samp in array"() -> (w563:i32)
        n206 = Reshape Array(w566, w563) -> (w564:dbl[])
        n207 = global read "effectiveglobals.vi" "PoreADCDT"() -> (w551:dbl)
        n208 = Index Array(array=w564, index=6) -> (element=w550:dbl)
        n209 = Subtract(x=w551, y=w550) -> (x-y=w546:dbl)
        n210 = Multiply(x=w546, y=0.025511) -> (x*y=w544:dbl)
        n211 = Absolute Value(x=w544) -> (abs(x)=w543:dbl)
        n212 = Multiply(x=0.005067074 ("y"), y=w543) -> (x*y=w557:dbl)
        n213 = global read "effectiveglobals.vi" "DeltaP"() -> (w554:dbl)
        n214 = Multiply(x=0.000889 ("y"), y=w557) -> (x*y=w559:dbl)
        n215 = global read "effectiveglobals.vi" "Thickness"() -> (w548:dbl)
        n216 = Multiply(x=w548, y=0.05) -> (x*y=w547:dbl)
        n217 = Multiply(x=w547, y=w559) -> (x*y=w556:dbl)
        n218 = Divide(x=w556, y=0.0049) -> (x/y=w553:dbl)
        n219 = Divide(x=w553, y=w554) -> (x/y=w552:dbl)
      }
      frame "Pore pressure A" {
        n220 = global read "effectiveglobals.vi" "Pressure A"() -> (w568:dbl)
      }
      frame "Pore pressure difference" {
        n221 = global read "effectiveglobals.vi" "DeltaP"() -> (w569:dbl)
      }
      frame "Porosity", Default {
        n222 = global read "effectiveglobals.vi" "Porosity"() -> (w570:dbl)
      }
      frame "Pore Pressure B displacement" {
        n223 = global read "effectiveglobals.vi" "PoreBDCDT"() -> (w571:dbl)
      }
      frame "Pore Pressure B" {
        n224 = global read "effectiveglobals.vi" "Pressure B"() -> (w572:dbl)
      }
    }
    n225 = case shown="True" "Zero y-axis" {
      tunnel: w389 -> [_ w593]
      tunnel: [w592 w593] -> w391
      tunnel: w390 -> [w592 _]
      frame False {
      }
      frame True {
      }
    }
    n226 = feedback-in #5(w391) -> ()
    n227 = Decrement(x=w518) -> (x-1=w505:i32)
    n228 = feedback #10() -> (w465:i32)  [unwired: 1 in]
    "Zeroed at:" <- w465
    n229 = case shown="True" "Zero Confine" {
      tunnel: [w607 w609] -> w466
      tunnel: [w606 w608] -> w467
      tunnel: w464 -> [w606 _]
      tunnel: w465 -> [w607 _]
      frame False {
      }
      frame True {
        n230 = global read "BiaxGlobals (16chan).vi" "Samp in array"() -> (w609:i32)
        n231 = global read "effectiveglobals.vi" "Confine"() -> (w608:dbl)
      }
    }
    n232 = feedback-in #7(w467) -> ()
    n233 = feedback-in #10(w466) -> ()
    n234 = feedback #11() -> (w476:i32)  [unwired: 1 in]
    "Zeroed at:" <- w476
    n235 = case shown="True" "Zero Normal" {
      tunnel: [w613 w615] -> w477
      tunnel: [w612 w614] -> w478
      tunnel: w474 -> [w612 _]
      tunnel: w476 -> [w613 _]
      frame False {
      }
      frame True {
        n236 = global read "BiaxGlobals (16chan).vi" "Samp in array"() -> (w615:i32)
        n237 = global read "effectiveglobals.vi" "NorLoad"() -> (w614:dbl)
      }
    }
    n238 = feedback-in #1(w478) -> ()
    n239 = feedback-in #11(w477) -> ()
    n240 = Equal To 0?(x=w505) -> (x = 0?=w530:bool)
    n241 = Subtract(x=w415, y=w414) -> (x-y=w413:dbl)
    n242 = global write "effectiveglobals.vi" "Zero x"(w384) -> ()
    n243 = feedback #12() -> (w379:dbl)  [unwired: 1 in]
    "Offset Voltage 2" <- w379
    n244 = case shown="True" "Offset X-axis 2" {
      tunnel: [w588 w589] -> w386
      tunnel: w379 -> [w588 _]
      tunnel: w372 -> [_ w589]
      frame False {
      }
      frame True {
      }
    }
    n245 = feedback-in #12(w386) -> ()
    n246 = global read "effectiveglobals.vi" "NorLoad"() -> (w473:dbl)
    n247 = Multiply "V to mm"(x=w413, y=0.766283524) -> (x*y=w426:dbl)
    n248 = global read "effectiveglobals.vi" "Confine"() -> (w463:dbl)
    n249 = global read "effectiveglobals.vi" "Pore A"() -> (w435:dbl)
    n250 = global read "effectiveglobals.vi" "Pore B"() -> (w432:dbl)
    n251 = Subtract(x=w473, y=w474) -> (x-y=w471:dbl)
    n252 = feedback #13() -> (w380:dbl)  [unwired: 1 in]
    "Offset Voltage 1" <- w380
    n253 = global write "effectiveglobals.vi" "offset x1"(w380) -> ()
    n254 = case shown="True" "Offset X-axis 1" {
      tunnel: [w590 w591] -> w383
      tunnel: w380 -> [w590 _]
      tunnel: w381 -> [_ w591]
      frame False {
      }
      frame True {
      }
    }
    n255 = feedback-in #13(w383) -> ()
    n256 = Multiply "mm to cm"(x="Thickness (2 layers, mm)", y=0.1 ("Thickness (2 layers, mm)")) -> (x*y=w369:dbl)
    n257 = Subtract(x=w463, y=w464) -> (x-y=w462:dbl)
    n258 = Subtract(x=w435, y=w356) -> (x-y=w434:dbl)
    n259 = Multiply "mm to cm"(x=w426, y=0.1) -> (x*y=w422:dbl)
    n260 = Subtract(x=w432, y=w355) -> (x-y=w431:dbl)
    n261 = case shown="True" "Horizontal Load" {
      tunnel: [52.91005291 5.501669757] -> w472
      frame False {
      }
      frame True {
      }
    }
    n262 = global read "BiaxGlobals (16chan).vi" "stop"() -> (w531:bool)
    n263 = Multiply "V to MPa"(x=6.752194463, y=w462) -> (x*y=w460:dbl)
    n264 = Subtract(x=w376, y=w384) -> (x-y=w402:dbl)
    n265 = Multiply "V to kN"(x=w472, y=w471) -> (x*y=w470:dbl)
    n266 = Subtract(x=w369, y=w422) -> (x-y=w409:dbl)
    n267 = global write "effectiveglobals.vi" "Thickness"(w369) -> ()
    n268 = Multiply(x=w434, y=6.816632584) -> (x*y=w433:dbl)
    n269 = Multiply(x=w431, y=6.788866259) -> (x*y=w430:dbl)
    n270 = Add(x=w402, y=w380) -> (x+y=w378:dbl)
    n271 = Subtract(x="Sample\n Area (m2)", y=w458) -> (x-y=w456:dbl)
    n272 = Divide(x=1.0, y="Calibration x-axis (V/unit)") -> (x/y=w397:dbl)
    n273 = Multiply "MPa to Pa"(x=w460, y=1000000.0) -> (x*y=w457:dbl)
    n274 = Divide "Volume of material"(x="Amount of material (g)", y="Material density (g/cm3)") -> (x/y=w419:dbl)
    n275 = Add(x=w378, y=w379) -> (x+y=w377:dbl)
    n276 = Multiply "kN to N"(x=w470, y=1000.0) -> (x*y=w455:dbl)
    n277 = Subtract(x=w389, y=w390) -> (x-y=w403:dbl)
    n278 = Multiply ("Total gouge volume")(x="Sample\n Area (m2)", y=10000.0) -> (x*y=w410:dbl)
    n279 = Multiply "Total gouge volume"(x=w410, y=w409) -> (x*y=w354:dbl)
    n280 = global read "BiaxGlobals (16chan).vi" "Var Rec Rate"() -> (w525:i32)
    "Record rate (samp/s)" <- w525
    n281 = Decrement(x=w525) -> (x-1=w524:i32)
    n282 = Array Subset(array=w506, index (row)=w524, length (row)=1, index (col)=0, length (col)=w516) -> (w527:dbl[][])
    n283 = global write "BiaxGlobals (16chan).vi" "stop"("stop") -> ()
    n284 = Multiply(x=w457, y=w456) -> (x*y=w454:dbl)
    n285 = Add(x=w354, y=3.8998) -> (x+y=w353:dbl)
    n286 = Reshape Array(w527, w510) -> (w514:dbl[])
    n287 = Add "Sigma_n = (FHP+Pc(A-Ap))/A"(x=w455, y=w454) -> (x+y=w453:dbl)
    n288 = Subtract(x=w353, y=w419) -> (x-y=w418:dbl)
    n289 = Add(x=w433, y=w430) -> (x+y=w441:dbl)
    n290 = call "BiaxXsig process (16chan).vi"("voltage data"=w514, "Numeric"=w511, "error in (no error)"=w513) -> ("AUX8"=w483:dbl, "AUX9"=w482:dbl, "Hor LVDT"=w493:dbl, "AUX7"=w484:dbl, "AUX6"=w485:dbl, "AUX5"=w486:dbl, "error out"=w512:errorcluster, "AUX12"=w481:dbl, "AUX4"=w487:dbl, "AUX11"=w479:dbl, "AUX10"=w480:dbl, "Hor Load"=w494:dbl, "Vert Load"=w491:dbl, "Ver LVDT"=w492:dbl, "AUX1"=w490:dbl, "AUX2"=w489:dbl, "AUX3"=w488:dbl)  [unwired: 7 in, 1 out]
    "Hor LVDT" <- w493
    "Hor Load (ch0)" <- w494
    "Vert Load (ch2)" <- w491
    "Vert LVDT (ch3)" <- w492
    "AUX1 (ch4)" <- w490
    "AUX2 (ch5)" <- w489
    "AUX3 (ch6)" <- w488
    "AUX4 (ch7)" <- w487
    "AUX5 (ch8)" <- w486
    "AUX6 (ch9)" <- w485
    "AUX7 (ch10)" <- w484
    "AUX8 (ch11)" <- w483
    "AUX9 (ch12)" <- w482
    "AUX10 (ch13)" <- w480
    "AUX11 (ch14)" <- w479
    "AUX12 (ch15)" <- w481
    n291 = Unbundle By Name(w512) -> ("status"=w533:bool)
    n292 = Not Or(1:w533, 2:w531) -> (0:w534:bool)
    n293 = global read "effectiveglobals.vi" "Pore B"() -> (w358:dbl)
    n294 = global read "effectiveglobals.vi" "Pore A"() -> (w363:dbl)
    n295 = Multiply(x=w377, y=w397) -> (x*y=w407:dbl)
    n296 = global write "effectiveglobals.vi" "AUX12(ch15)"(w481) -> ()
    n297 = global write "effectiveglobals.vi" "PoreBDCDT"(w486) -> ()
    n298 = Divide(x=w453, y="Sample\n Area (m2)") -> (x/y=w452:dbl)
    n299 = Divide ("material")(x=w418, y=w353) -> (x/y=w417:dbl)
    n300 = feedback #14() -> (w507:i32)  [unwired: 1 in]
    n301 = case shown="True" w530 {
      tunnel: w504 -> [w718 w728]
      tunnel: w509 -> [w717 w729]
      tunnel: w538 -> [w716 w725]
      tunnel: [w716 w724] -> w537
      tunnel: w512 -> [w715 w726]
      tunnel: [w715 w723] -> w536
      tunnel: [w712 i16[][] []] -> w535
      tunnel: [w711 w720] -> w508
      tunnel: w507 -> [w711 _]
      frame False {
        n302 = Build Array (concatenate)(w717, w718) -> (w712:i32[][])
        n303 = global read "BiaxGlobals (16chan).vi" "Countdown"() -> (w714:i32)
        n304 = Decrement(x=w714) -> (x-1=w713:i32)
        n305 = global write "BiaxGlobals (16chan).vi" "Countdown"(w713) -> ()
      }
      frame True {
        n306 = Build Array (concatenate)(w729, w728) -> (w722:i32[][])
        n307 = Write to Binary File(file (use dialog)=w725, data=w722, error in=w726, 5:FALSE ("prepend array or string size? (T)"), 9:T2."native, host order" ("byte order (0:big-endian, network order)")) -> (refnum out=w724:refnum<file>, error out=w723:errorcluster)  [unwired: 1 in, 1 out]
        n308 = global read "BiaxGlobals (16chan).vi" "Sample write number"() -> (w733:i16)
        n309 = global read "BiaxGlobals (16chan).vi" "Time interval to write to disk (s)"() -> (w730:i32)
        "Write countdown" <- w730
        n310 = Increment(x=w733) -> (x+1=w727:i16)
        n311 = Multiply(x=w727, y=w730) -> (x*y=→"Time into data acq. (s)":i32)
        n312 = global read "BiaxGlobals (16chan).vi" "Samp in array"() -> (w720:i32)
        "Saved sample No." <- w720
        n313 = global write "BiaxGlobals (16chan).vi" "Sample write number"(w727) -> ()
        n314 = global write "BiaxGlobals (16chan).vi" "Countdown"(w730) -> ()
      }
    }
    n315 = feedback-in #14(w508) -> ()
    n316 = Subtract(x=w358, y=w355) -> (x-y=w357:dbl)
    n317 = global write "effectiveglobals.vi" "PoreADCDT"(w488) -> ()
    n318 = global write "effectiveglobals.vi" "AUX7(ch10)"(w484) -> ()
    n319 = global write "effectiveglobals.vi" "VerDCDT"(w492) -> ()
    n320 = Subtract(x=w363, y=w356) -> (x-y=w362:dbl)
    n321 = Divide(x=w357, y=0.1473) -> (x/y=w359:dbl)
    n322 = global write "effectiveglobals.vi" "AUX9(ch12)"(w482) -> ()
    n323 = Multiply ("Total gouge volume")(x=w417, y=100.0 ("x*y")) -> (x*y=w385:dbl)
    "Porosity (%)" <- w385
    n324 = Divide(x=w441, y=2.0) -> (x/y=w437:dbl)
    "Average Pore pressure" <- w437
    n325 = Divide(x=1.0, y="Calibration y-axis (V/unit)") -> (x/y=w394:dbl)
    n326 = Multiply(x=w403, y=w394) -> (x*y=w370:dbl)
    n327 = call "XY.vi"("Enable"="Show plot", "Reset"="Reset plot", "Y Input"=w370, "X Input"=w407) -> ("XY Graph"=→"XY plot":cluster{"Y":dbl[], "Y":dbl[]}[])  [unwired: 6 in, 1 out]
    n328 = Divide(x=w362, y=0.1467) -> (x/y=w360:dbl)
    n329 = global write "effectiveglobals.vi" "NorDcDT"(w493) -> ()
    n330 = global write "effectiveglobals.vi" "ConfDCDT"(w490) -> ()
    n331 = global write "effectiveglobals.vi" "Porosity"(w385) -> ()
    n332 = Subtract(x=w360, y=w359) -> (x-y=w368:dbl)
    n333 = Divide "Pa to MPa"(x=w452, y=1000000.0) -> (x/y=w439:dbl)
    n334 = global write "effectiveglobals.vi" "Pressure B"(w359) -> ()
    n335 = global write "effectiveglobals.vi" "Pressure A"(w360) -> ()
    n336 = Subtract(x=w439, y=w437) -> (x-y=→"Effective normal \nstress (MPa)":dbl)
    n337 = Absolute Value(x=w368) -> (abs(x)=w367:dbl)
    n338 = global write "effectiveglobals.vi" "Ver LOAD"(w491) -> ()
    n339 = Multiply(x=1000000.0, y=w367) -> (x*y=w365:dbl)
    n340 = global write "effectiveglobals.vi" "Aux10(ch13)"(w480) -> ()
    n341 = global write "effectiveglobals.vi" "AUX11CH14)"(w479) -> ()
    n342 = global write "effectiveglobals.vi" "Pore B"(w485) -> ()
    n343 = global write "effectiveglobals.vi" "NorLoad"(w494) -> ()
    n344 = global write "effectiveglobals.vi" "AUX8(ch11)"(w483) -> ()
    n345 = global write "effectiveglobals.vi" "Pore A"(w487) -> ()
    n346 = global write "effectiveglobals.vi" "Confine"(w489) -> ()
    n347 = global write "effectiveglobals.vi" "DeltaP"(w365) -> ()
  }
  n348 = Number To Decimal String(number=w78) -> (decimal integer string=w77:string)  [unwired: 1 in]
  n349 = Concatenate Strings(w77, "                " ("string")) -> (w75:string)
  n350 = String Subset(string=w75, length (rest)=16 ("length (rest)")) -> (substring=w73:string)  [unwired: 1 in]
  n351 = call <vilib>:"DAQmx Clear Task.vi"("task in"=w20, "error in"=w22) -> ("error out"=w24:errorcluster)  [unwired: 13 in]
  n352 = Concatenate Strings(w72, w73, w71) -> (w66:string)
  n353 = case shown="True" w70 {
    tunnel: [w735 w739] -> w68
    tunnel: w69 -> [w735 w740]
    tunnel: w67 -> [w734 w737]
    tunnel: [w734 w738] -> w17
    tunnel: w66 -> [_ w736]
    frame False {
    }
    frame True {
      n354 = Write to Text File(file (use dialog)=w740, text=w736, error in=w737) -> (refnum out=w739:refnum<file>, error out=w738:errorcluster)  [unwired: 1 in, 1 out]
    }
  }
  n355 = Merge Errors(w18, w17) -> (w16:errorcluster)
  n356 = call <vilib>:"DAQmx Clear Task.vi"("task in"=w21, "error in"=w16) -> ("error out"=w19:errorcluster)  [unwired: 13 in]
  n357 = Merge Errors(w19, w24) -> (w23:errorcluster)
  n358 = call <vilib>:"Close File+.vi"("error in (no error)"=w17, "refnum"=w68) -> ()  [unwired: 3 in, 3 out]
  n359 = call <vilib>:"Simple Error Handler.vi"("type of dialog (OK msg:1)"=w25, "error in (no error)"=w23) -> ()  [unwired: 3 in, 5 out]
  "Processor scan rate" <- w30
